vi "XYVoltageToMeters.vi"(8 "error in (no error)":errorcluster, 9 "Y Voltage":dbl, 10 "X Voltage":dbl, 11 "Asylum_Driver in":refnum<class "Asylum_Driver.lvclass">) -> (0 "error out":errorcluster, 1 "Y Meters":dbl, 2 "X Meters":dbl, 3 "Asylum_Driver out":refnum<class "Asylum_Driver.lvclass">)   [LabVIEW 2019, in "Asylum_Driver.lvclass"]
uses:
  Asylum_Driver.lvclass
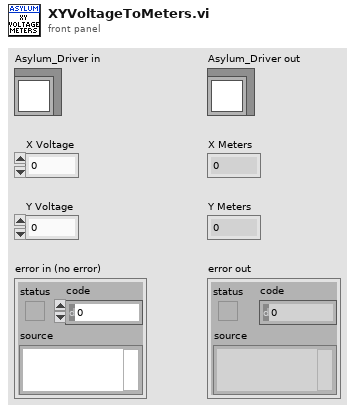
[diagram p1: front panel]
types:
  T1 = cluster{"XLVDT Sens":dbl, "YLVDT Sens":dbl, "XLVDT Offset":dbl, "YLVDT Offset":dbl}
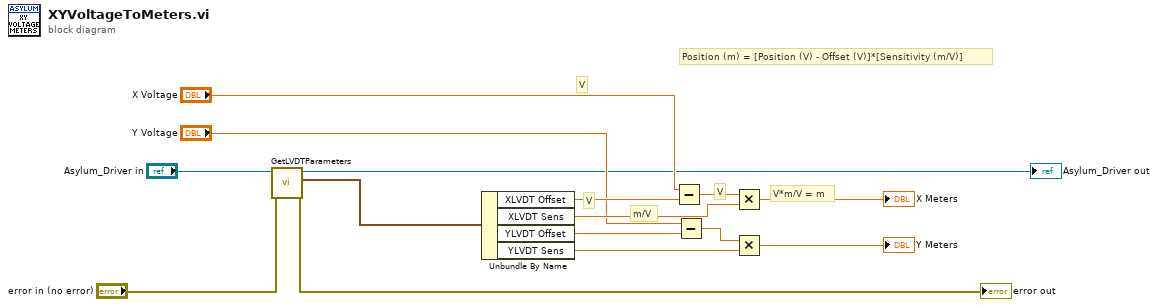
[diagram p0: block diagram]
diagram:
  # "Position (m) = [Position (V) - Offset (V)]*[Sensitivity (m/V)]"
  # "m/V"
  # "V*m/V = m"
  # "V"
  # "V"
  # "V"
  n1 = call "GetLVDTParameters.vi"("error in (no error)"="error in (no error)", "Asylum_Driver in"="Asylum_Driver in") -> ("error out"=→"error out":errorcluster, "LVDT Parameters"=w3:T1, "Asylum_Driver out"=→"Asylum_Driver out":refnum<class "Asylum_Driver.lvclass">)  [unwired: 7 in]
  n2 = Unbundle By Name(w3) -> ("XLVDT Offset"=w10:dbl, "XLVDT Sens"=w12:dbl, "YLVDT Offset"=w15:dbl, "YLVDT Sens"=w14:dbl)
  n3 = Subtract(x="X Voltage", y=w10) -> (x-y=w11:dbl)
  n4 = Subtract(x="Y Voltage", y=w15) -> (x-y=w13:dbl)
  n5 = Multiply(x=w11, y=w12) -> (x*y=→"X Meters":dbl)
  n6 = Multiply(x=w13, y=w14) -> (x*y=→"Y Meters":dbl)
